vi "UI Manager Proxy_Create.vi"(0 "reference in":refnum<class "UI Manager Proxy.lvclass">, 5 "Error In":errorcluster) -> (14 "reference out":refnum<class "UI Manager Proxy.lvclass">, 19 "Error Out":errorcluster)   [LabVIEW 2024, in "UI Manager Proxy.lvclass"]
uses:
  UI Manager Proxy.lvclass
  C:/Users/burakkorkmaz/Desktop/Leveling/labview-desing-patterns/Proxy Pattern/User Manager_class/User Manager.lvclass
  UI Manager Proxy.lvclass/UI Manager Proxy.ctl
  User Manager_class/User Manager.lvclass
  UI Manager_class/UI Manager.lvclass
  C:/Users/burakkorkmaz/Desktop/Leveling/labview-desing-patterns/Proxy Pattern/UI Manager Proxy_class/UI Manager Proxy.lvclass
panel:
  # "Connector Pane"
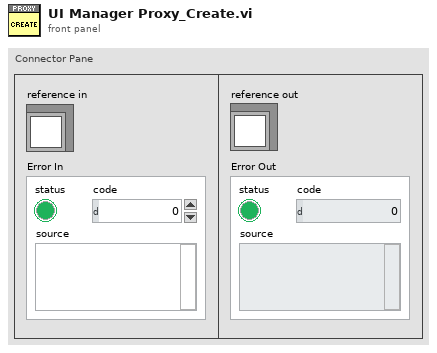
[diagram p1: front panel]
types:
  T1 = typedef "UI Manager Proxy.lvclass/ObjectAttributes.ctl" = cluster{"UI Manager":refnum<class "UI Manager.lvclass">, "UserLevel":T2}
  T2 = typedef "UserLevel.ctl" = enum16{"System Manager", "Admin", "Operator"}
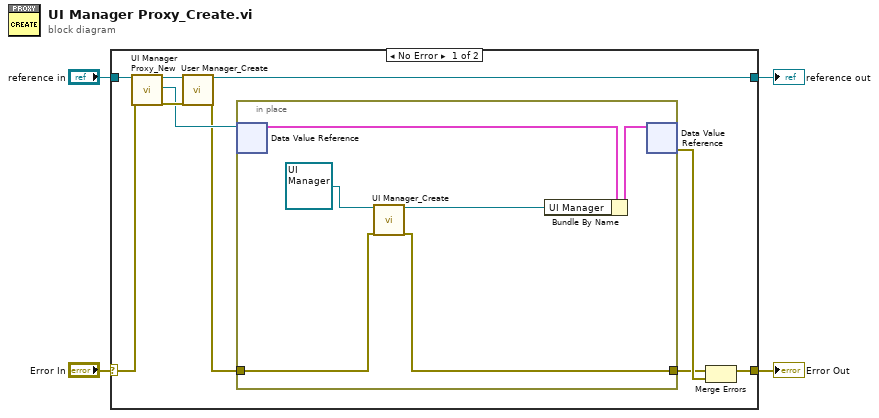
[diagram p0: block diagram]
diagram:
  n1 = case shown="No Error" "Error In" {
    selector: "Error In" -> [w13 w22]
    tunnel: [w11 w22] -> w3
    tunnel: "reference in" -> [w14 w21]
    tunnel: [w8 w21] -> w1
    frame No Error {
      n2 = call "UI Manager Proxy_New.vi"("reference in"=w14, "Error In"=w13) -> ("reference out"=w10:refnum<class "UI Manager Proxy.lvclass">, "DVRRefOut"=w7:refnum<data-value>, "Error Out"=w9:errorcluster)  [unwired: 14 in, 1 out]
      n3 = call "User Manager_Create.vi"("reference in"=w10, "Error In"=w9) -> ("reference out"=w8:refnum<class "UI Manager Proxy.lvclass">, "Error Out"=w6:errorcluster)  [unwired: 16 in]
      n4 = in-place {
        in-place-border: w6 -> [w17]
        in-place-border: [w16] -> w5
        n5 = in-place-dvr #1(w7) -> (w19:T1)  [unwired: 1 out]
        n6 = call "UI Manager_Create.vi"("reference in"=refnum<class "UI Manager.lvclass"> refnum ("UI Manager"), "Error In"=w17) -> ("reference out"=w15:refnum<class "UI Manager.lvclass">, "Error Out"=w16:errorcluster)  [unwired: 16 in]
        n7 = Bundle By Name(cluster=w19, "UI Manager"=w15) -> (w20:T1)
        n8 = in-place-dvr #1(w20) -> (w12:errorcluster)  [unwired: 1 out]
      }
      n9 = Merge Errors(w5, w12) -> (w11:errorcluster)
    }
    frame Error {
    }
  }
  "Error Out" <- w3
  "reference out" <- w1
